vi "GetTargetBuildSpecs.vi"(8 "error in (no error)":errorcluster, 9 "Name of target (My Computer)":string="My Computer", 10 "Name of build specification (if empty: get all)":string, 11 "Path to project":path) -> (0 "error out":errorcluster, 2 "buildspec refs":refnum<vi>[](array[refnum]), 3 "project ref":refnum<vi>)   [LabVIEW 2020]
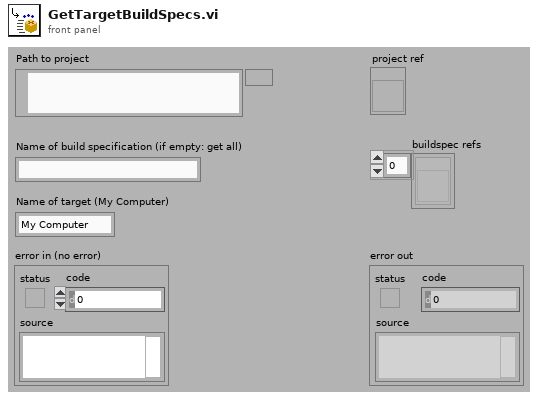
[diagram p1: front panel]
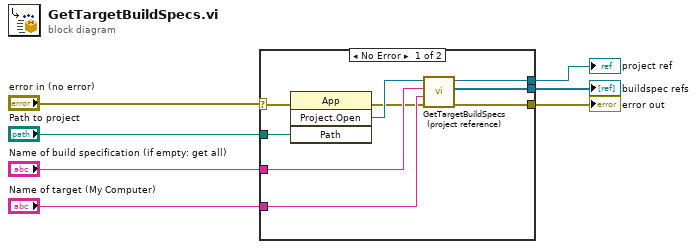
[diagram p0: block diagram]
diagram:
  n1 = case shown="No Error" "error in (no error)" {
    selector: "error in (no error)" -> [w15 w17]
    tunnel: "Path to project" -> [w16 _]
    tunnel: "Name of target (My Computer)" -> [w13 _]
    tunnel: "Name of build specification (if empty: get all)" -> [w12 _]
    tunnel: [w8 w17] -> w4
    tunnel: [w11 _] -> w1
    tunnel: [w9 _] -> w2
    frame No Error {
      n2 = invoke class="App" method="Project.Open"(error in=w15, "Path"=w16) -> (error out=w10:errorcluster, "Project:Open"=w14:refnum<vi>)  [unwired: 2 in, 2 out]
      n3 = call <vilib>:"GetTargetBuildSpecs (project reference).vi"("error in (no error)"=w10, "Name of target (My Computer)"=w13, "Name of build specification (if empty: get all)"=w12, "Project reference"=w14) -> ("error out"=w8:errorcluster, "buildspec refs"=w9:refnum<vi>[], "project ref"=w11:refnum<vi>)  [unwired: 5 in]
    }
    frame Error {
    }
  }
  "error out" <- w4
  "buildspec refs" <- w2
  "project ref" <- w1
